vi "AlazarConfigureLSB.vi"(3 "error in (no error)":errorcluster, 4 "Value LSB 1":u32, 5 "Value LSB 0":u32, 6 "Handle":u64) -> (0 "error out":errorcluster, 1 "Return Code":u32, 2 "Handle":u64)   [LabVIEW 2009]
doc: "12- and 14-bit digitzers return 16-bit sample values with sample codes stored in the most-significant bits of each 16-bit sample value. By default, the least-significant bits of each sample value are zero filled. Use this option to used these otherwise unused bits as digital outputs."
uses:
  ATSApi.dll
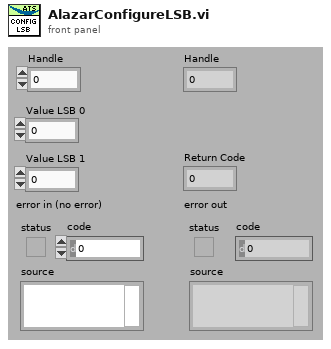
[diagram p1: front panel]
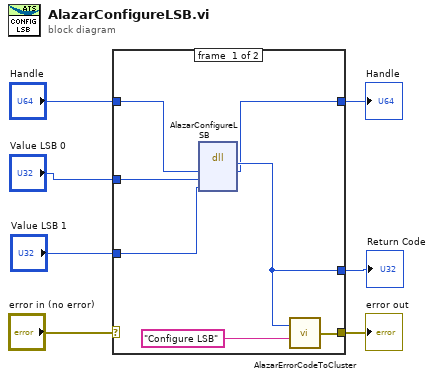
[diagram p0: block diagram]
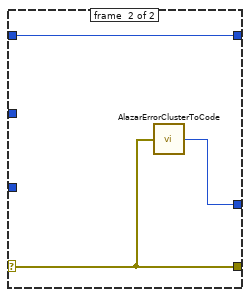
[diagram p2: hidden frame]
diagram:
  n1 = case shown="No Error" "error in (no error)" {
    selector: "error in (no error)" -> [_ w17]
    tunnel: [w11 w17] -> w6
    tunnel: [w13 w16] -> w5
    tunnel: "Handle" -> [w14 w15]
    tunnel: [w10 w15] -> w3
    tunnel: "Value LSB 0" -> [w9 _]
    tunnel: "Value LSB 1" -> [w8 _]
    frame #0 {
      n2 = dll-call lib="ATSApi.dll" fn="AlazarConfigureLSB"("handle"=w14, "valueLsb0"=w9, "valueLsb1"=w8) -> ("return type"=w13:u32, "handle"=w10:u64)  [unwired: 5 in, 2 out]
      n3 = call "AlazarErrorCodeToCluster.vi"("Message"="Configure LSB", "Error Code"=w13) -> ("error out"=w11:errorcluster)
    }
    frame #1 {
      n4 = call "AlazarErrorClusterToCode.vi"("error in (no error)"=w17) -> ("Error Code"=w16:u32)
    }
  }
  "Handle" <- w3
  "error out" <- w6
  "Return Code" <- w5
